vi "PiColorStrings.vi"(10 "String":string, 11 "String in":refnum<vi>) -> (3 "String out":refnum<vi>)   [LabVIEW 2019]
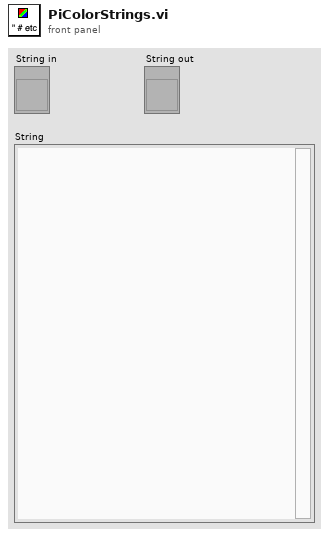
[diagram p1: front panel]
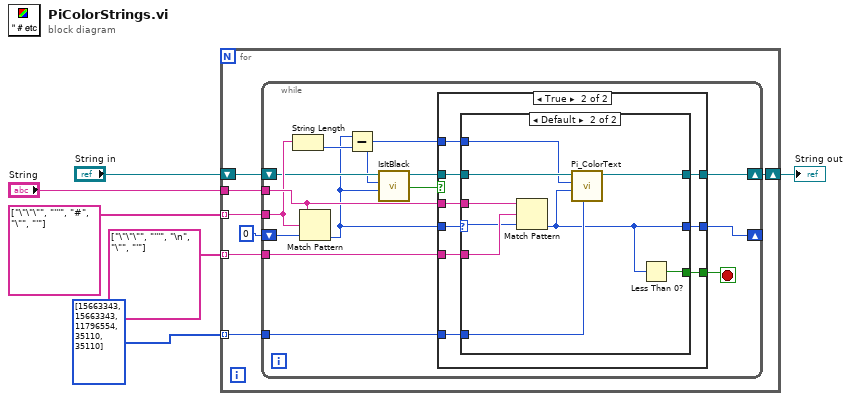
[diagram p0: block diagram]
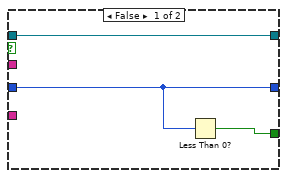
[diagram p2: hidden frame]
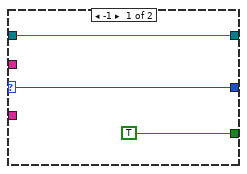
[diagram p3: hidden frame]
diagram:
  n1 = for {
    shift-right: [w12] -> w5
    shift-left: "String in" -> [w13]
    tunnel: string[] ["\"\"\"", "'''", "#", "\"", "'"] -> [w9] mode=indexing
    tunnel: "String" -> [w11]
    tunnel: string[] ["\"\"\"", "'''", "\n", "\"", "'"] -> [w8] mode=indexing
    tunnel: u32[] [15663343, 15663343, 11796554, 35110, 35110] -> [w7] mode=indexing
    n2 = while {
      tunnel: w11 -> [w24]
      tunnel: w9 -> [w20]
      shift-right: [w27] -> w12
      shift-left: w13 -> [w19]
      shift-right: [w21] -> _
      shift-left: 0 -> [w25]
      tunnel: w8 -> [w23]
      tunnel: w7 -> [w22]
      stop <- w26 stop-if-true
      n3 = String Length(string=w20) -> (length=w18:i32)
      n4 = Match Pattern(string=w24, regular expression=w20, offset (0)=w25) -> (offset past match=w16:i32)  [unwired: 3 out]
      n5 = Subtract(x=w16, y=w18) -> (x-y=w17:i32)
      n6 = call "IsItBlack.vi"("End"=w16, "Start"=w17, "String in"=w19) -> ("Black?"=w14:bool, "String out"=w15:refnum<vi>)  [unwired: 7 in]
      n7 = case shown="True" w14 {
        tunnel: [w30 w39] -> w27
        tunnel: [w28 w38] -> w26
        tunnel: w24 -> [_ w37]
        tunnel: w23 -> [_ w36]
        tunnel: w22 -> [_ w35]
        tunnel: [w29 w34] -> w21
        tunnel: w15 -> [w30 w33]
        tunnel: w17 -> [_ w32]
        tunnel: w16 -> [w29 w31]
        frame False {
          n8 = Less Than 0?(x=w29) -> (x < 0?=w28:bool)
        }
        frame True {
          n9 = case shown="Default" w31 {
            selector: w31 -> [w40 w45]
            tunnel: w33 -> [w41 w51]
            tunnel: [w41 w50] -> w39
            tunnel: [TRUE ("Text.Font:Bold") w46] -> w38
            tunnel: w37 -> [_ w49]
            tunnel: w36 -> [_ w48]
            tunnel: w35 -> [_ w47]
            tunnel: [w40 w43] -> w34
            tunnel: w32 -> [_ w44]
            frame -1 {
            }
            frame Default {
              n10 = Match Pattern(string=w49, regular expression=w48, offset (0)=w45) -> (offset past match=w43:i32)  [unwired: 3 out]
              n11 = call "Pi_ColorText.vi"("Color"=w47, "End"=w43, "Start"=w44, "String in"=w51) -> ("String out"=w50:refnum<vi>)  [unwired: 7 in]
              n12 = Less Than 0?(x=w43) -> (x < 0?=w46:bool)
            }
          }
        }
      }
    }
  }
  "String out" <- w5
